vi "Get Angle.vi"(6 "Axis":T1, 8 "error in (no error)":errorcluster, 11 "Inst.Xeryon-Rotator in":refnum<class "Inst.Xeryon-Rotator.lvclass">) -> (0 "error out":errorcluster, 1 "Status":string, 2 "Angle (°)":dbl, 3 "Inst.Xeryon-Rotator out":refnum<class "Inst.Xeryon-Rotator.lvclass">)   [LabVIEW 2019, in "Inst.Xeryon-Rotator.lvclass"]
uses:
  Inst.Xeryon-Rotator.lvclass
  C:/Program Files (x86)/National Instruments/LabVIEW 2019/user.lib/LevyLab/Instrument Framework/Instrument/Instrument.lvclass
  <userlib>/LevyLab/Instrument Framework/Instrument Types/Cryostat/Typedefs/Rotator Axis--Enum.ctl
  Typedefs/Inst.Xeryon-Rotator.Commands--Enum.ctl
  773e2a9d-0901-4956-ae6e-010e7225b876.vi
  773e2a9d-0901-4956-ae6e-010e7225b876.vi/11828800-3453-4f84-86bd-3e81b3592072.vi
  773e2a9d-0901-4956-ae6e-010e7225b876.vi/0ca54dff-c6eb-4130-ae76-37ac1b1013e3.vi
  <vilib>/Utility/Data Type/Get Type Information.vi
  <vilib>/JDP Science/JSONtext/JSON text to Variant.vi
  <vilib>/JDP Science/JSONtext/LVClass Serializer/JSONtext LVClass Serializer.lvclass
  <userlib>/LevyLab/Instrument Framework/Instrument/Instrument.lvclass
  <userlib>/LevyLab/Instrument Framework/Instrument Types/Cryostat/Typedefs/getAngle--cluster.ctl
  <userlib>/LevyLab/Instrument Framework/Instrument Types/Cryostat/Instrument.Cryostat.lvclass
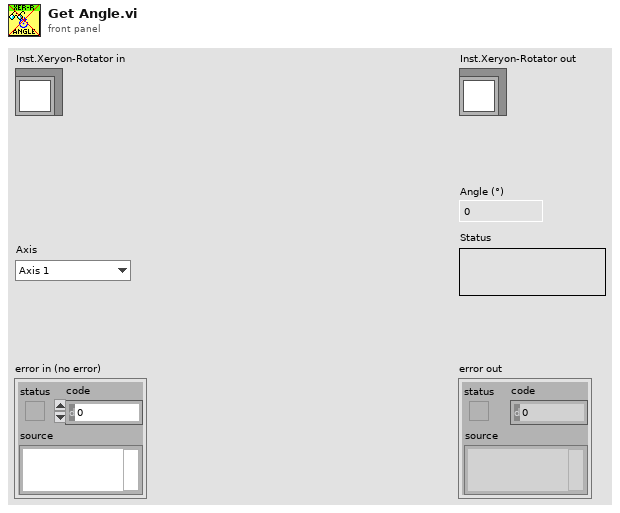
[diagram p1: front panel]
types:
  T1 = typedef "Instrument.Cryostat.lvclass/Rotator Axis--Enum.ctl" = enum16{"Axis 1", "Axis 2"}
  T2 = typedef "Instrument.Cryostat.lvclass/getAngle--cluster.ctl" = cluster{"angle":dbl, "status":string, "finished":bool}
  T3 = typedef "Inst.Xeryon-Rotator.lvclass/Inst.Xeryon-Rotator.Commands--Enum.ctl" = enum16{"setAngle", "getAngle", "setState"}
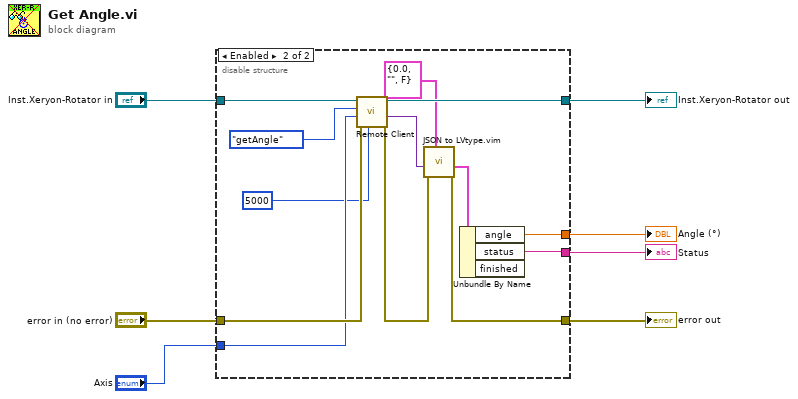
[diagram p0: block diagram]
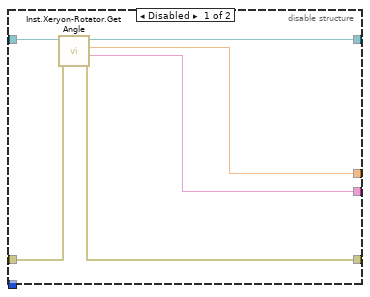
[diagram p2: hidden frame]
diagram:
  n1 = disable-structure shown="Enabled" {
    disable-tunnel: "Inst.Xeryon-Rotator in" -> [w13 w26]
    disable-tunnel: [w12 w25] -> w6
    disable-tunnel: [w11 w14] -> w5
    disable-tunnel: "error in (no error)" -> [w10 w21]
    disable-tunnel: [w9 w22] -> w3
    disable-tunnel: [w8 w23] -> w2
    disable-tunnel: "Axis" -> [_ w20]
    frame Disabled {
      n2 = call "Inst.Xeryon-Rotator.Get Angle.vi"("error in (no error)"=w10, "Inst.Xeryon-Rotator in"=w13) -> ("error out"=w11:errorcluster, "delimited string"=w9:string, "EPOS In Current Units"=w8:dbl, "Inst.Xeryon-Rotator out"=w12:refnum<class "Inst.Xeryon-Rotator.lvclass">)  [unwired: 6 in]
    }
    frame Enabled {
      n3 = call <userlib>:"Remote Client.vi"("timeout (ms) [500]"=5000, "error in (no error)"=w21, "Data in"=w20, "Command in"=Inst.Xeryon-Rotator.Commands--Enum."getAngle" ("Commands"), "Instrument in"=w26) -> ("error out"=w15:errorcluster, "Data out"=w17:variant, "Instrument out"=w25:refnum<class "Inst.Xeryon-Rotator.lvclass">)  [unwired: 3 in, 1 out]
      n4 = call "JSON to LVtype.vim"("type"=T2 {"angle"=0.0, "status"="", "finished"=FALSE} ("getAngle"), "error in (no error)"=w15, "JSON Data in"=w17) -> ("error out"=w14:errorcluster, "Data out"=w16:T2)  [unwired: 7 in]
      n5 = Unbundle By Name(w16) -> ("angle"=w23:dbl, "status"=w22:string)  [unwired: 1 out]
    }
  }
  "error out" <- w5
  "Inst.Xeryon-Rotator out" <- w6
  "Angle (°)" <- w2
  "Status" <- w3
